vi "New-Window.vi"(8 "error in (no error)":errorcluster) -> (0 "error out":errorcluster, 3 "Window out":refnum<class "Window.lvclass">)   [LabVIEW 2024, in "GLF.lvlib" / "Window.lvclass"]
uses:
  Window.lvclass
  Window.lvclass/Window.ctl
  DVR--cluster.ctl
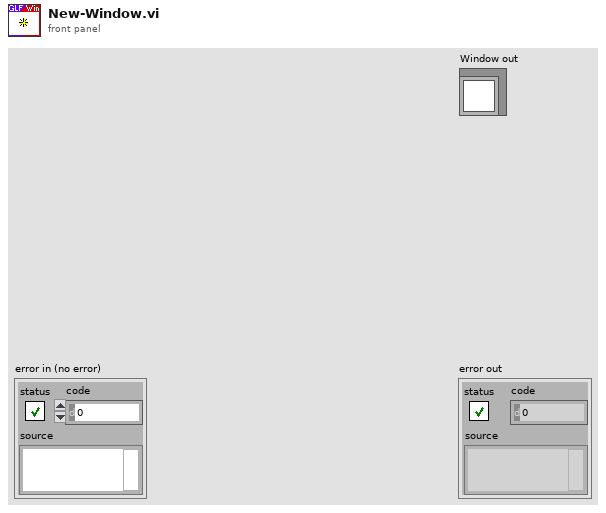
[diagram p1: front panel]
types:
  T1 = typedef "GLF.lvlib/Window.lvclass/DVR--cluster.ctl" = cluster{"foo":dbl}
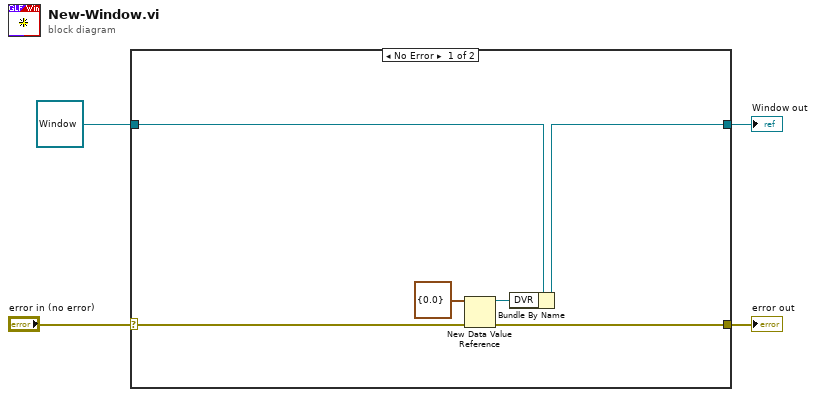
[diagram p0: block diagram]
diagram:
  n1 = case shown="No Error" "error in (no error)" {
    selector: "error in (no error)" -> [w9 w12]
    tunnel: [w8 w12] -> w3
    tunnel: [w6 w11] -> w1
    tunnel: refnum<class "Window.lvclass"> refnum ("Window in") -> [w10 w11]
    frame No Error {
      n2 = New Data Value Reference(data value=T1 {"foo"=0.0} ("DVR"), error in=w9) -> (data value reference=w5:refnum<data-value>, error out=w8:errorcluster)
      n3 = Bundle By Name(cluster=w10, "DVR"=w5) -> (w6:refnum<class "Window.lvclass">)
    }
    frame Error {
    }
  }
  "error out" <- w3
  "Window out" <- w1
